vi "RTS Station Setup Settings.vi"(8 "Error In":errorcluster, 9 "TDMS Data Save Input":T1, 10 "Data":T3={"Clients"=[], "Listener"=refnum, "Data Array"=["1-1 PF C:\\Technology Lab\\NI-2010\\Trunk\\Refrigeration\\RTS\\Old System\\Point\\16P00290.Pnt"]}, 11 "RTS Config Setup Input":T4) -> (0 "Error Out":errorcluster, 1 "TDMS Data Save Output":T1, 3 "RTS Config Setup Output":T4)   [LabVIEW 2016]
uses:
  Type Definitions/RTS Configuration Setup.ctl
  Type Definitions/RTS Wago Config.ctl
  Type Definitions/RTS APLUS Config.ctl
  Type Definitions/RTS Yokogawa MX Config.ctl
  Type Definitions/RTS Replay Server Control.ctl
  Type Definitions/RTS Server Configuration.ctl
  Type Definitions/RTS Station Settions TCP Comms.ctl
  Type Definitions/RTS Chamber Save Status.ctl
  Type Definitions/RTS Test Pattern.ctl
  Type Definitions/RTS TCP Multiple Connections Data.ctl
  Type Definitions/RTS TDMS Filename Locations.ctl
  Type Definitions/RTS Save References.ctl
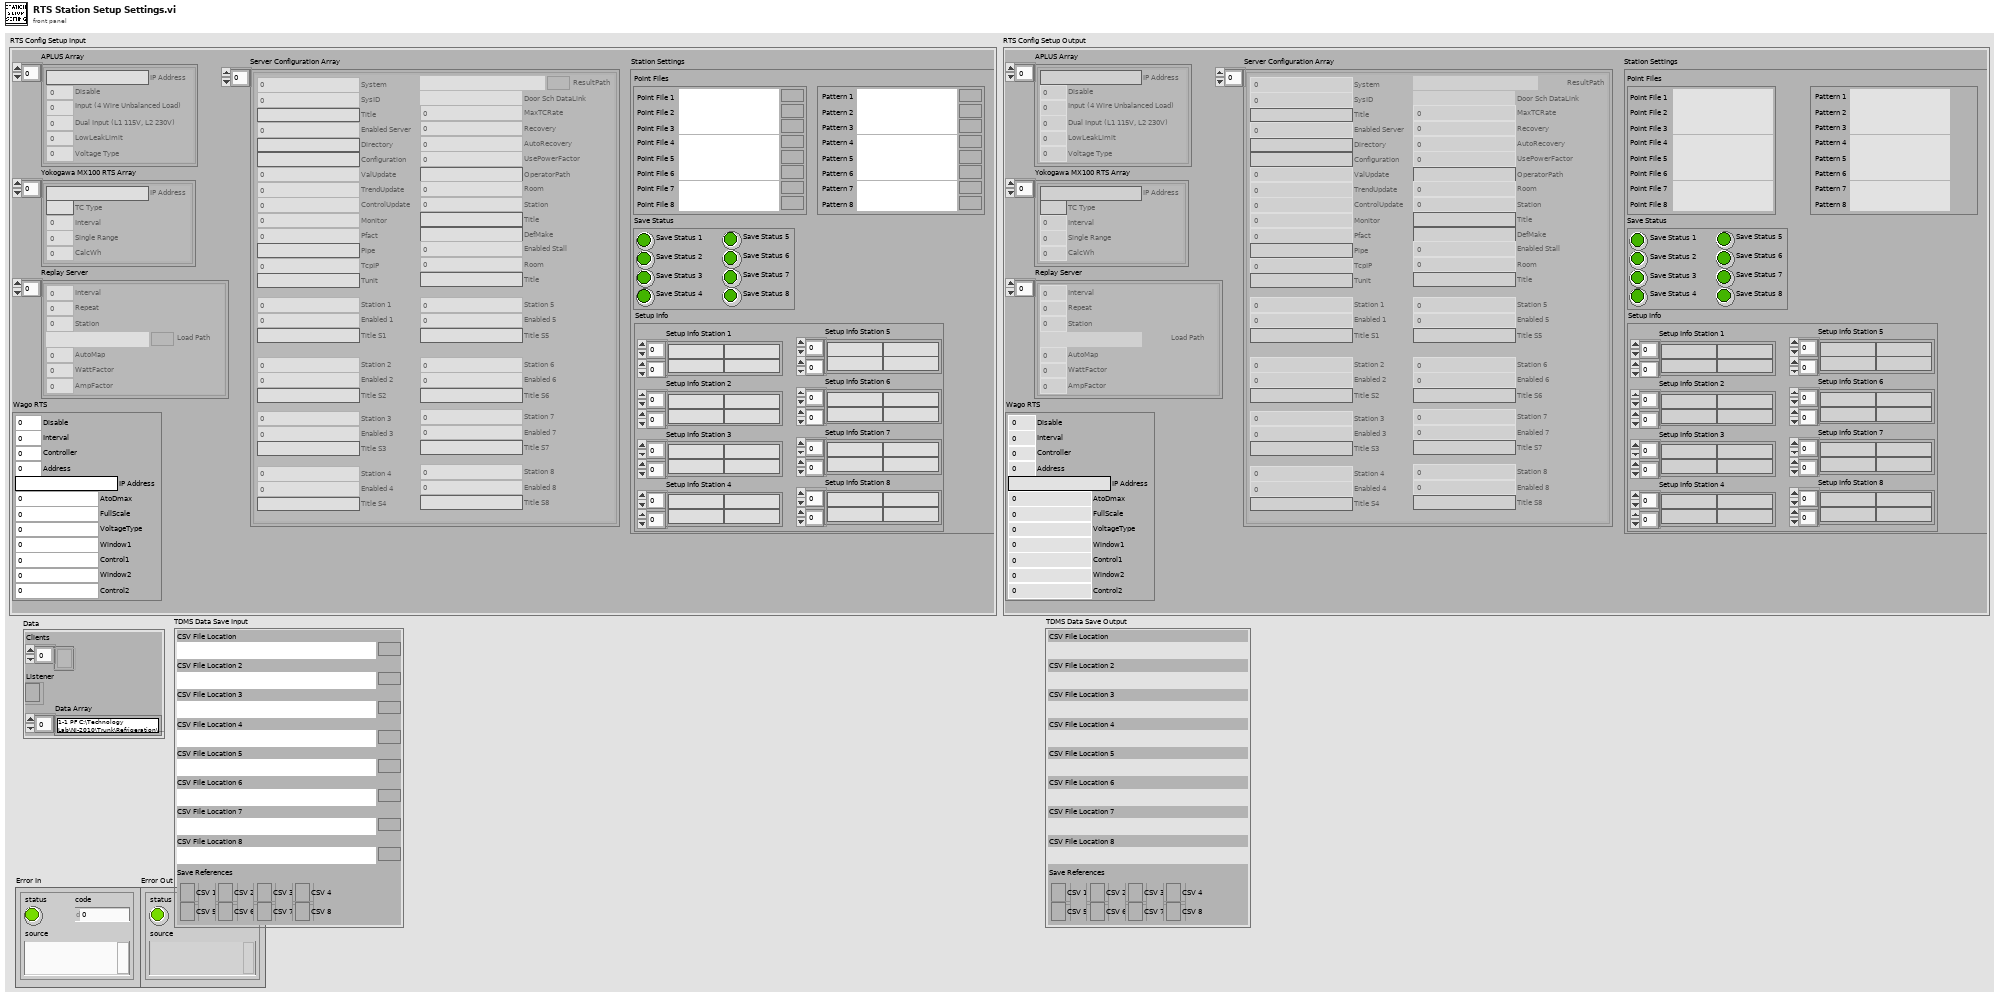
[diagram p1: front panel]
types:
  T1 = typedef "RTS TDMS Filename Locations.ctl" = cluster{"CSV File Location":path, "CSV File Location 2":path, "CSV File Location 3":path, "CSV File Location 4":path, "CSV File Location 5":path, "CSV File Location 6":path, "CSV File Location 7":path, "CSV File Location 8":path, "Save References":T2}
  T2 = typedef "RTS Save References.ctl" = cluster{"CSV 1":refnum<file>, "CSV 2":refnum<file>, "CSV 3":refnum<file>, "CSV 4":refnum<file>, "CSV 5":refnum<file>, "CSV 6":refnum<file>, "CSV 7":refnum<file>, "CSV 8":refnum<file>}
  T3 = typedef "RTS TCP Multiple Connections Data.ctl" = cluster{"Clients":refnum<k5>[], "Listener":refnum<k5>, "Data Array":string[]}
  T4 = typedef "RTS Configuration Setup.ctl" = cluster{"Wago RTS":T5, "APLUS Array":T6[], "Yokogawa MX100 RTS Array":T7[], "Replay Server":T8[], "Server Configuration Array":T9[], "Station Settings":T10}
  T5 = typedef "RTS Wago Config.ctl" = cluster{"Disable":u16, "Interval":u16, "Controller":u16, "Address":u16, "IP Address":string, "AtoDmax":u16, "FullScale":u16, "VoltageType":u16, "Window1":u16, "Control1":u16, "Window2":u16, "Control2":u16}
  T6 = typedef "RTS APLUS Config.ctl" = cluster{"Disable":u16, "IP Address":string, "Input (4 Wire Unbalanced Load)":u16, "Dual Input (L1 115V, L2 230V)":u16, "LowLeakLimit":dbl, "Voltage Type":u16}
  T7 = typedef "RTS Yokogawa MX Config.ctl" = cluster{"IP Address":string, "TC Type":string, "Interval":u16, "Single Range":u16, "CalcWh":u16}
  T8 = typedef "RTS Replay Server Control.ctl" = cluster{"Interval":i16, "Repeat":u16, "Station":u16, "Load Path":path, "AutoMap":u16, "WattFactor":dbl, "AmpFactor":dbl}
  T9 = typedef "RTS Server Configuration.ctl" = cluster{"System":u16, "SysID":u16, "Title":string, "Enabled Server":u16, "Directory":string, "Configuration":string, "ValUpdate":u16, "TrendUpdate":u16, "ControlUpdate":u16, "Monitor":u16, "Pfact":u16, "Pipe":string, "TcpIP":u16, "Tunit":string, "ResultPath":path, "Door Sch DataLink":path, "MaxTCRate":u16, "Recovery":u16, "AutoRecovery":u16, "UsePowerFactor":u16, "OperatorPath":string, "Room":u16, "Station":u16, "Title":string, "DefMake":string, "Enabled Stall":u16, "Room":u16, "Title":string, "Station 1":u16, "Enabled 1":u16, "Station 2":u16, "Enabled 2":u16, "Station 3":u16, "Enabled 3":u16, "Station 4":u16, "Enabled 4":u16, "Station 5":u16, "Enabled 5":u16, "Station 6":u16, "Enabled 6":u16, "Station 7":u16, "Enabled 7":u16, "Station 8":u16, "Enabled 8":u16, "Title S1":string, "Title S2":string, "Title S3":string, "Title S5":string, "Title S6":string, "Title S7":string, "Title S8":string, "Title S4":string}
  T10 = typedef "RTS Station Settions TCP Comms.ctl" = cluster{"Point Files":cluster{"Point File 1":path, "Point File 2":path, "Point File 3":path, "Point File 4":path, "Point File 5":path, "Point File 6":path, "Point File 7":path, "Point File 8":path}, "Save Status":T11, "Setup Info":cluster{"Setup Info Station 1":string[][], "Setup Info Station 2":string[][], "Setup Info Station 3":string[][], "Setup Info Station 4":string[][], "Setup Info Station 5":string[][], "Setup Info Station 6":string[][], "Setup Info Station 7":string[][], "Setup Info Station 8":string[][]}, "Chamber Test Pattern":T12}
  T11 = typedef "RTS Chamber Save Status.ctl" = cluster{"Save Status 1":bool, "Save Status 2":bool, "Save Status 3":bool, "Save Status 4":bool, "Save Status 5":bool, "Save Status 6":bool, "Save Status 7":bool, "Save Status 8":bool}
  T12 = typedef "RTS Test Pattern.ctl" = cluster{" Pattern 1":path, "Pattern 2":path, "Pattern 3":path, "Pattern 4":path, "Pattern 5":path, "Pattern 6":path, "Pattern 7":path, "Pattern 8":path}
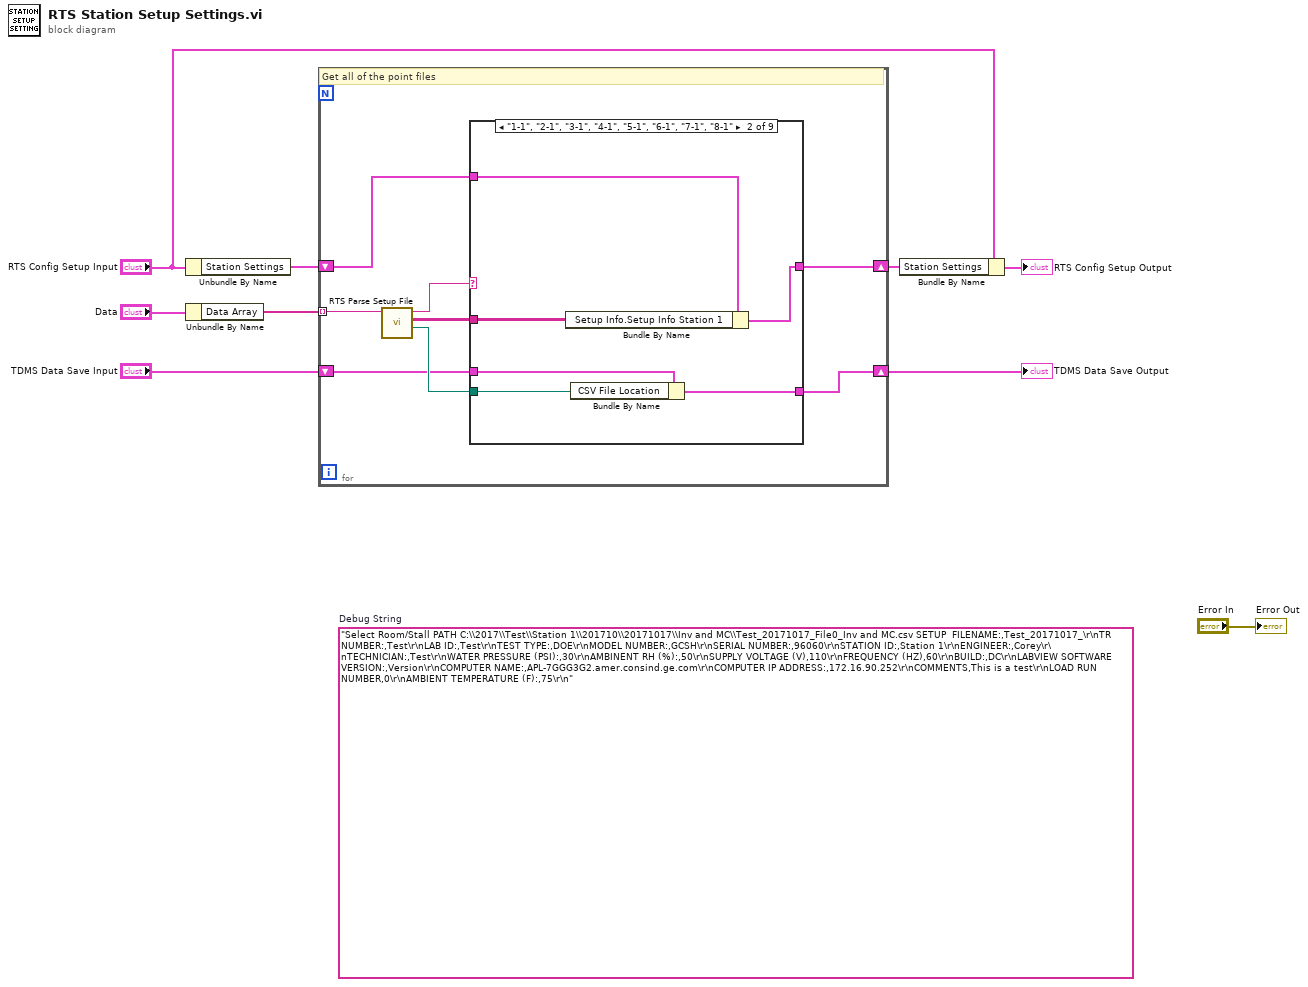
[diagram p0: block diagram]
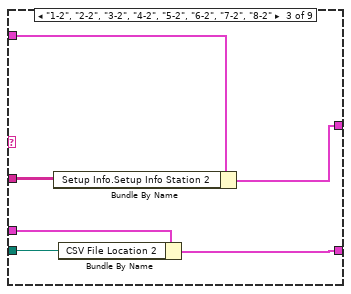
[diagram p3: hidden frame]
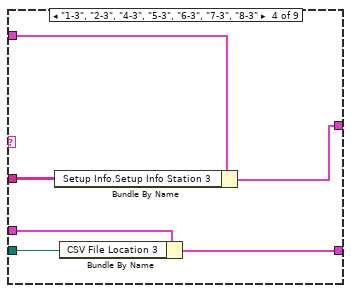
[diagram p4: hidden frame]
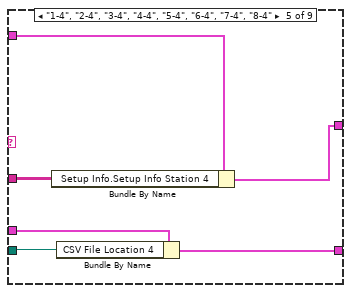
[diagram p5: hidden frame]
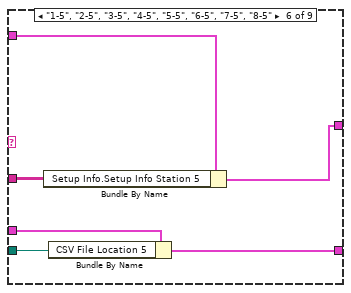
[diagram p6: hidden frame]
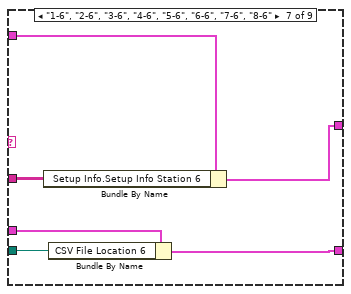
[diagram p7: hidden frame]
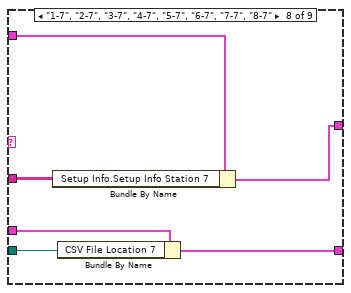
[diagram p8: hidden frame]
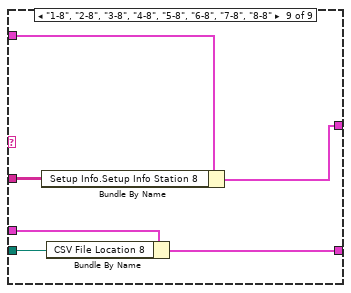
[diagram p9: hidden frame]
diagram:
  (unwired) "Select Room/Stall PATH C:\\2017\\Test\\Station 1\\201710\\20171017\\Inv and MC\\Test_20171017_File0_Inv and MC.csv SETUP  FILENAME:,Test_20171017_\r\nTR NUMBER:,Test\r\nLAB ID:,Test\r\nTEST TYPE:,DOE\r\nMODEL NUMBER:,GCSH\r\nSERIAL NUMBER:,96060\r\nSTATION ID:,Station 1\r\nENGINEER:,Corey\r\nTECHNICIAN:,Test\r\nWATER PRESSURE (PSI):,30\r\nAMBINENT RH (%):,50\r\nSUPPLY VOLTAGE (V),110\r\nFREQUENCY (HZ),60\r\nBUILD:,DC\r\nLABVIEW SOFTWARE VERSION:,Version\r\nCOMPUTER NAME:,APL-7GGG3G2.amer.consind.ge.com\r\nCOMPUTER IP ADDRESS:,172.16.90.252\r\nCOMMENTS,This is a test\r\nLOAD RUN NUMBER,0\r\nAMBIENT TEMPERATURE (F):,75\r\n"  # Debug String
  n1 = Unbundle By Name("RTS Config Setup Input") -> ("Station Settings"=w3:T10)
  n2 = Unbundle By Name("Data") -> ("Data Array"=w8:string[])
  n3 = for {
    tunnel: w8 -> [w17] mode=indexing
    shift-right: [w12] -> w4
    shift-left: w3 -> [w15]
    shift-right: [w10] -> w1
    shift-left: "TDMS Data Save Input" -> [w11]
    # "Get all of the point files"
    n4 = call "RTS Parse Setup File.vi"("Data"=w17) -> ("Save Path"=w13:path, "Setup Info Station 8"=w14:string[][], "Station ID"=w16:string)  [unwired: 8 in]
    n5 = case shown="\"1-1\", \"2-1\", \"3-1\", \"4-1\", \"5-1\", \"6-1\", \"7-1\", \"8-1\"" w16 {
      tunnel: w15 -> [w19 w25 w31 w37 w43 w49 w55 w61 w67]
      tunnel: [w19 w24 w30 w36 w42 w48 w54 w60 w66] -> w12
      tunnel: w14 -> [_ w23 w29 w35 w41 w47 w53 w59 w65]
      tunnel: w13 -> [_ w21 w26 w32 w38 w44 w50 w56 w62]
      tunnel: w11 -> [w18 w22 w28 w34 w40 w46 w52 w58 w64]
      tunnel: [w18 w20 w27 w33 w39 w45 w51 w57 w63] -> w10
      frame Default {
      }
      frame "1-1", "2-1", "3-1", "4-1", "5-1", "6-1", "7-1", "8-1" {
        n6 = Bundle By Name(cluster=w25, "Setup Info.Setup Info Station 1"=w23) -> (w24:T10)
        n7 = Bundle By Name(cluster=w22, "CSV File Location"=w21) -> (w20:T1)
      }
      frame "1-2", "2-2", "3-2", "4-2", "5-2", "6-2", "7-2", "8-2" {
        n8 = Bundle By Name(cluster=w31, "Setup Info.Setup Info Station 2"=w29) -> (w30:T10)
        n9 = Bundle By Name(cluster=w28, "CSV File Location 2"=w26) -> (w27:T1)
      }
      frame "1-3", "2-3", "4-3", "5-3", "6-3", "7-3", "8-3" {
        n10 = Bundle By Name(cluster=w37, "Setup Info.Setup Info Station 3"=w35) -> (w36:T10)
        n11 = Bundle By Name(cluster=w34, "CSV File Location 3"=w32) -> (w33:T1)
      }
      frame "1-4", "2-4", "3-4", "4-4", "5-4", "6-4", "7-4", "8-4" {
        n12 = Bundle By Name(cluster=w43, "Setup Info.Setup Info Station 4"=w41) -> (w42:T10)
        n13 = Bundle By Name(cluster=w40, "CSV File Location 4"=w38) -> (w39:T1)
      }
      frame "1-5", "2-5", "3-5", "4-5", "5-5", "6-5", "7-5", "8-5" {
        n14 = Bundle By Name(cluster=w49, "Setup Info.Setup Info Station 5"=w47) -> (w48:T10)
        n15 = Bundle By Name(cluster=w46, "CSV File Location 5"=w44) -> (w45:T1)
      }
      frame "1-6", "2-6", "3-6", "4-6", "5-6", "6-6", "7-6", "8-6" {
        n16 = Bundle By Name(cluster=w55, "Setup Info.Setup Info Station 6"=w53) -> (w54:T10)
        n17 = Bundle By Name(cluster=w52, "CSV File Location 6"=w50) -> (w51:T1)
      }
      frame "1-7", "2-7", "3-7", "4-7", "5-7", "6-7", "7-7", "8-7" {
        n18 = Bundle By Name(cluster=w61, "Setup Info.Setup Info Station 7"=w59) -> (w60:T10)
        n19 = Bundle By Name(cluster=w58, "CSV File Location 7"=w56) -> (w57:T1)
      }
      frame "1-8", "2-8", "3-8", "4-8", "5-8", "6-8", "7-8", "8-8" {
        n20 = Bundle By Name(cluster=w67, "Setup Info.Setup Info Station 8"=w65) -> (w66:T10)
        n21 = Bundle By Name(cluster=w64, "CSV File Location 8"=w62) -> (w63:T1)
      }
    }
  }
  "TDMS Data Save Output" <- w1
  n22 = Bundle By Name(cluster="RTS Config Setup Input", "Station Settings"=w4) -> (→"RTS Config Setup Output":T4)
  "Error Out" <- "Error In"
